vi "PWM Configuration to Channel Settings.vi"(6 "PWM":T1 {"PWM Channels"."PWM frequency" items=["1 Hz", "50 Hz", "250 Hz", "500 Hz", "1 kHz", "5 kHz", "10 kHz", "20 kHz"]}, 8 "error in":errorcluster, 9 "default values":dbl[](array[numeric]), 10 "names":string[](array[string]), 11 "PWM Mode in":refnum<class "PWM Mode.lvclass">) -> (0 "error out":errorcluster, 2 "channel settings":T2[](array[typedef]), 3 "PWM Mode out":refnum<class "PWM Mode.lvclass">)   [LabVIEW 2017, in "Scan Engine Scripting.lvlib" / "PWM Mode.lvclass"]
uses:
  PWM Mode.lvclass
  Controls/pwm channel settings.ctl
  Channel Classes/PWM Output Channel/Frequency.ctl
  Channel Classes/PWM Output Channel/PWM Output Channel.lvclass
  Scan Engine Scripting.lvlib
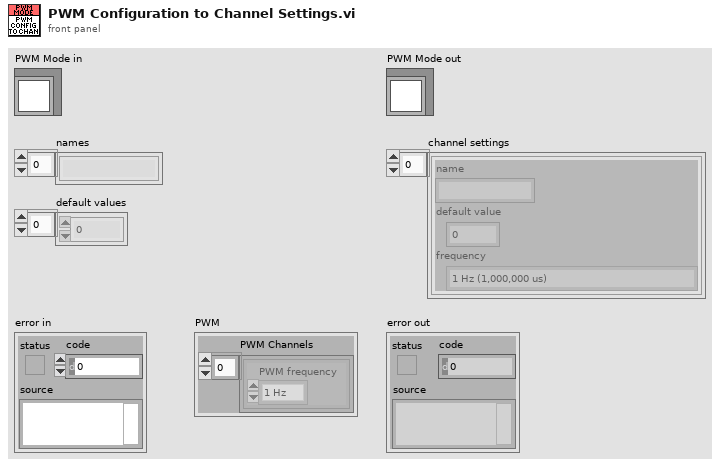
[diagram p1: front panel]
types:
  T1 = cluster{"PWM Channels":cluster{"PWM frequency":u32}[]}
  T2 = typedef "Scan Engine Scripting.lvlib/pwm channel settings.ctl" = cluster{"name":string, "default value":dbl, "frequency":T3}
  T3 = typedef "Scan Engine Scripting.lvlib/PWM Output Channel.lvclass/Frequency.ctl" = enum16{"1 Hz (1,000,000 us)", "50 Hz (20,000 us)", "250 Hz (4,000 us)", "500 Hz (2,000 us)", "1 kHz (1,000 us)", "5 kHz (200 us)", "10 kHz (100 us)", "20 kHz (50 us)"}
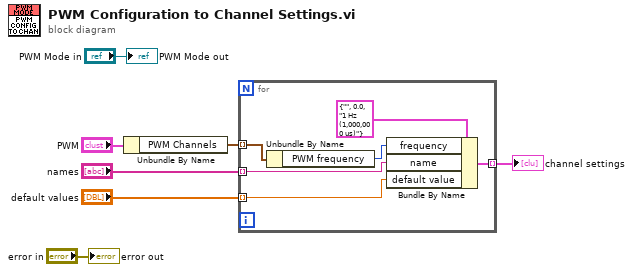
[diagram p0: block diagram]
diagram:
  n1 = Unbundle By Name("PWM") -> ("PWM Channels"=w7:cluster{"PWM frequency":u32}[])
  n2 = for {
    tunnel: w7 -> [w13] mode=indexing
    tunnel: "names" -> [w10] mode=indexing
    tunnel: "default values" -> [w9] mode=indexing
    tunnel: [w8] -> w2 mode=indexing
    n3 = Unbundle By Name(w13) -> ("PWM frequency"=w11:u32)
    n4 = Bundle By Name(cluster=T2 {"name"="", "default value"=0.0, "frequency"=enum."1 Hz (1,000,000 us)"} ("channel settings"), "frequency"=w11, "name"=w10, "default value"=w9) -> (w8:T2)
  }
  "channel settings" <- w2
  "error out" <- "error in"
  "PWM Mode out" <- "PWM Mode in"
